vi "SVT Decimated Exp Avg Level (1 Ch).vi"(6 "restart averaging (F)":bool, 7 "decimation factor":i32=-1, 8 "error in (no error)":errorcluster, 9 "time constant [ms]":dbl=125.0 format="%.2f", 10 "exponential mode":enum16{"Slow", "Fast", "Impulse", "Custom"}(ring)=enum."Fast", 11 "scaled signal [EU]":waveform(dbl)) -> (0 "error out":errorcluster, 1 "actual time constant [ms]":dbl=nan format="%.2f", 2 "unit label":string, 3 "decimated exp avg level [EU rms]":waveform(dbl), 5 "actual decimation factor":i32=-1)   [LabVIEW 2017]
doc: "Computes the exponential average level of <B>scaled signal [EU]</B> or <B>even angle signal [EU]</B> and then decimates the level signal by <B>decimation factor</B>. You can use this polymorphic VI to compute the exponential average level for a single channel or for N channels or for a single channel or N channels of angular resampled data. The data type you wire to the <B>scaled signal [EU]</B> or <B>even angle signal [EU]</B> input determines the polymorphic instance to use."
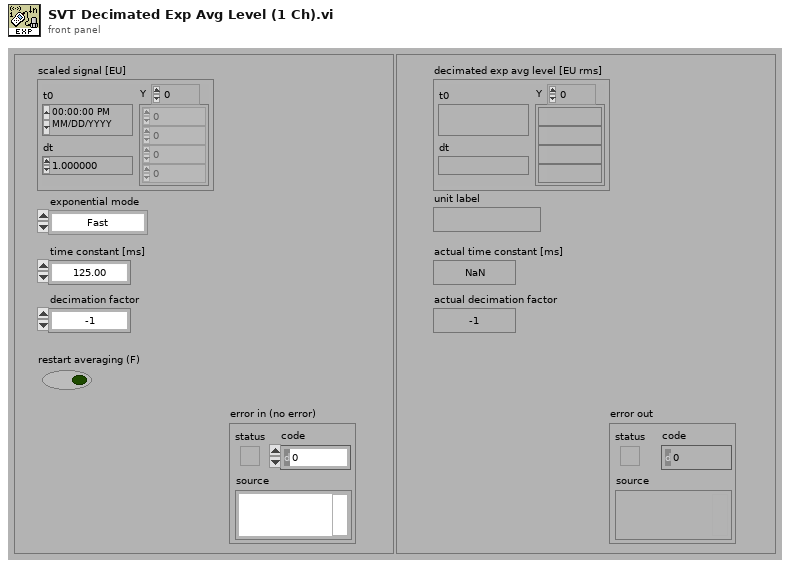
[diagram p1: front panel]
types:
  T1 = enum16{"RMS", "Running RMS", "Exp avg  ", "Dec exp avg ", "Peak", "Crest"}
  T2 = enum16{"Reset filter", "Restart averaging", "Continue processing"}
  T3 = typedef "svc_Channel Info.ctl" = cluster{"sensor sensitivity":dbl, "engineering units":T4, "dB reference":dbl, "custom label":string, "weighting filter":T5, "pregain":dbl}
  T4 = typedef "svc_Engineering Units Text Ring.ctl" = u16
  T5 = typedef "svc_Weighting Filter Text Ring.ctl" = u16
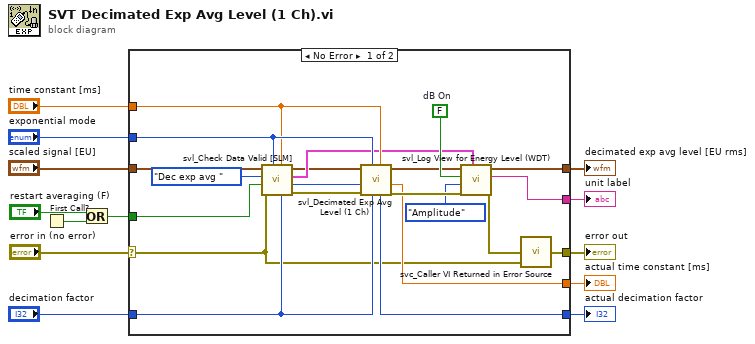
[diagram p0: block diagram]
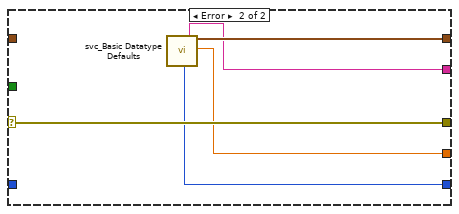
[diagram p2: hidden frame]
diagram:
  n1 = First Call?() -> (First Call?: T/F=w8:bool)
  n2 = Or(x="restart averaging (F)", y=w8) -> (x .or. y?=w7:bool)
  n3 = case shown="No Error" "error in (no error)" {
    tunnel: [w15 w38] -> w13
    tunnel: [w22 w39] -> w12
    tunnel: [w30 w35] -> w11
    tunnel: "scaled signal [EU]" -> [w18 _]
    tunnel: w7 -> [w21 _]
    tunnel: "exponential mode" -> [w26 _]
    tunnel: "time constant [ms]" -> [w25 _]
    tunnel: "decimation factor" -> [w20 _]
    tunnel: [w24 w36] -> w3
    tunnel: [w23 w37] -> w2
    selector: "error in (no error)" -> [w14 w39]
    frame No Error {
      w31 = FALSE  # dB On
      n4 = call <vilib>:"svl_Check Data Valid [SLM].vi"("decimation factor"=w20, "time constant [ms]"=w25, "exponential mode"=w26, "error in (no error)"=w14, "restart averaging (F)"=w21, "Level Analysis"=T1."Dec exp avg ", "scaled signal [EU]"=w18) -> ("error out"=w34:errorcluster, "processing state"=w27:T2, "channel info"=w17:T3, "dup scaled signal [EU]"=w16:waveform(dbl))  [unwired: 1 in]
      n5 = call <vilib>:"svl_Decimated Exp Avg Level (1 Ch).vi"("time constant [ms]"=w25, "decimation factor"=w20, "exponential mode"=w26, "error in (no error)"=w34, "processing state"=w27, "scaledSignal"=w16) -> ("error out"=w33:errorcluster, "actual time constant [ms]"=w23:dbl, "expAveragedArray"=w29:waveform(dbl), "actual decimation factor"=w24:i32)  [unwired: 2 in]
      n6 = call <vilib>:"svl_Log View for Energy Level (WDT).vi"("channel info"=w17, "error in (no error)"=w33, "view mode"=enum16{"Power", "Amplitude"}."Amplitude", "dB On (T)"=w31, "scaledSignal"=w29) -> ("error out"=w32:errorcluster, "unit label"=w30:string, "scaledSignal"=w15:waveform(dbl))  [unwired: 4 in]
      n7 = call <vilib>:"svc_Caller VI Returned in Error Source.vi"("warning input to caller"=w14, "error in (no error)"=w32) -> ("error out"=w22:errorcluster)  [unwired: 3 in]
    }
    frame Error {
      n8 = call <vilib>:"svc_Basic Datatype Defaults.vi"() -> ("zero I32"=w36:i32, "empty string"=w35:string, "empty waveform"=w38:waveform(dbl), "NaN"=w37:dbl)  [unwired: 7 in, 9 out]
    }
  }
  "unit label" <- w11
  "actual time constant [ms]" <- w2
  "decimated exp avg level [EU rms]" <- w13
  "error out" <- w12
  "actual decimation factor" <- w3
